vi "PF1.vi"(6 "错误输入（无错误）":errorcluster, 8 "error message":string, 10 "字符串":string, 11 "PF IN":refnum<vi>) -> (3 "引用输出":refnum<vi>, 4 "错误输出":errorcluster)   [LabVIEW 2018]
panel:
  out "UUTPF":string caption="UUT1PF"
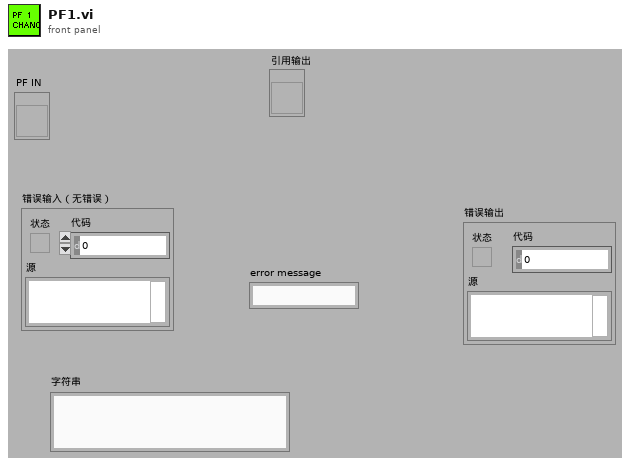
[diagram p1: front panel]
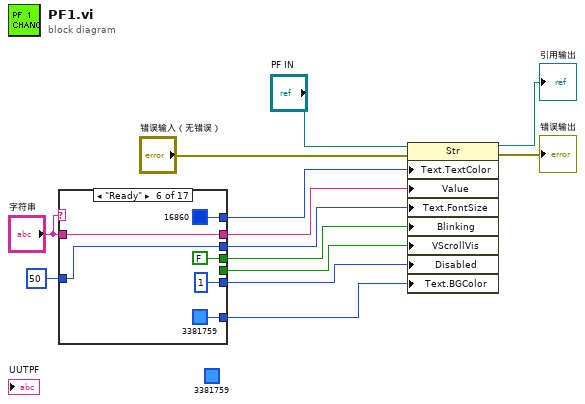
[diagram p0: block diagram]
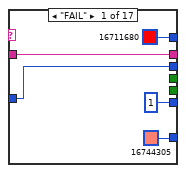
[diagram p2: hidden frame]
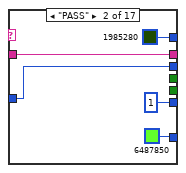
[diagram p3: hidden frame]
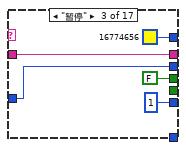
[diagram p4: hidden frame]
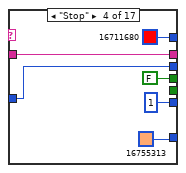
[diagram p5: hidden frame]
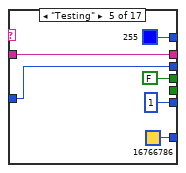
[diagram p6: hidden frame]
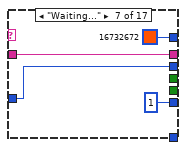
[diagram p7: hidden frame]
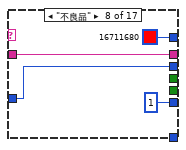
[diagram p8: hidden frame]
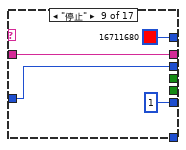
[diagram p9: hidden frame]
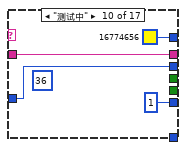
[diagram p10: hidden frame]
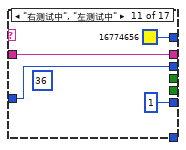
[diagram p11: hidden frame]
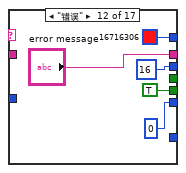
[diagram p12: hidden frame]
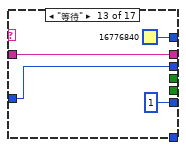
[diagram p13: hidden frame]
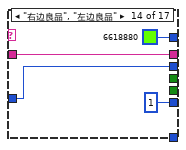
[diagram p14: hidden frame]
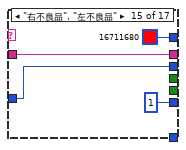
[diagram p15: hidden frame]
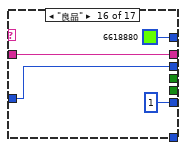
[diagram p16: hidden frame]
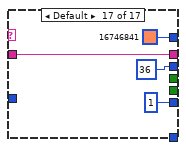
[diagram p17: hidden frame]
diagram:
  (unwired) u32 3381759
  n1 = case shown="\"Ready\"" "字符串" {
    tunnel: [u32 16711680 u32 1985280 u32 16774656 u32 16711680 u32 255 u32 16860 u32 16732672 u32 16711680 u32 16711680 u32 16774656 u32 16774656 u32 16716306 u32 16776840 u32 6618880 u32 16711680 u32 6618880 u32 16746841] -> w6
    tunnel: [_ _ FALSE FALSE FALSE FALSE _ _ _ _ _ _ _ _ _ _ _] -> w9
    tunnel: [w17 w22 w26 w32 w39 w45 w49 w54 w58 w62 w66 "error message" w75 w79 w83 w87 w90] -> w11
    tunnel: "字符串" -> [w17 w22 w26 w32 w39 w45 w49 w54 w58 w62 w66 _ w75 w79 w83 w87 w90]
    tunnel: [w15 w20 w24 w30 w36 w42 w47 w51 w55 w59 w63 u32 16 ("文本.字体:字号") w72 w76 w80 w84 u32 36 ("文本.字体:字号")] -> w8
    tunnel: [_ _ _ _ _ _ _ _ _ _ _ TRUE _ _ _ _ _] -> w5
    tunnel: [1 1 1 1 1 1 1 1 1 1 1 0 1 1 1 1 1] -> w4
    tunnel: u32 50 ("文本.字体:字号") -> [w15 w20 w24 w30 w36 w42 w47 w51 w55 w59 w63 _ w72 w76 w80 w84 _]
    tunnel: [u32 16744305 u32 6487850 _ u32 16755313 u32 16766786 u32 3381759 _ _ _ _ _ _ _ _ _ _ _] -> w1
    frame "FAIL" {
    }
    frame "PASS" {
    }
    frame "暂停" {
    }
    frame "Stop" {
    }
    frame "Testing" {
    }
    frame "Ready" {
    }
    frame "Waiting..." {
    }
    frame "不良品" {
    }
    frame "停止" {
    }
    frame "测试中" {
      (unwired) u32 36 ("文本.字体:字号")
    }
    frame "右测试中", "左测试中" {
      (unwired) u32 36 ("文本.字体:字号")
    }
    frame "错误" {
    }
    frame "等待" {
    }
    frame "右边良品", "左边良品" {
    }
    frame "右不良品", "左不良品" {
    }
    frame "良品" {
    }
    frame Default {
    }
  }
  n2 = property on="属性节点" class="Str"(reference="PF IN", error in="错误输入（无错误）", "Text.TextColor"=w6, "Value"=w11, "Text.FontSize"=w8, "Blinking"=w9, "VScrollVis"=w5, "Disabled"=w4, "Text.BGColor"=w1) -> (reference out=→"引用输出":refnum<vi>, error out=→"错误输出":errorcluster)
